vi "Populate Ctrl.vi"(8 "error in (no error)":errorcluster, 11 "FK Field in":refnum<class "FK Field.lvclass">) -> (0 "error out":errorcluster, 3 "FK Field out":refnum<class "FK Field.lvclass">)   [LabVIEW 2020, in "Composed Fields.lvlib" / "FK Field.lvclass"]
uses:
  FK Field.lvclass
  C:/Users/User/Documents/LabVIEW Code/LV-Database-OOP/source/Database OOP/Column Libraries/Column/Composed Column.lvclass
  Ring Ctrl Value Source/Ring Ctrl Value Source.lvclass
  Column/Composed Column.lvclass/Composed Column.ctl
  Composed Columns/Value Source Interface Class/Value Source.lvclass
  Basic Columns/Column Configuration/Basic Column Configuration Class/Column Configuration.lvclass
  Database Libraries/Database Interfaces/Database Interface Class/Database Interface.lvclass
  Column/Composed Column.lvclass
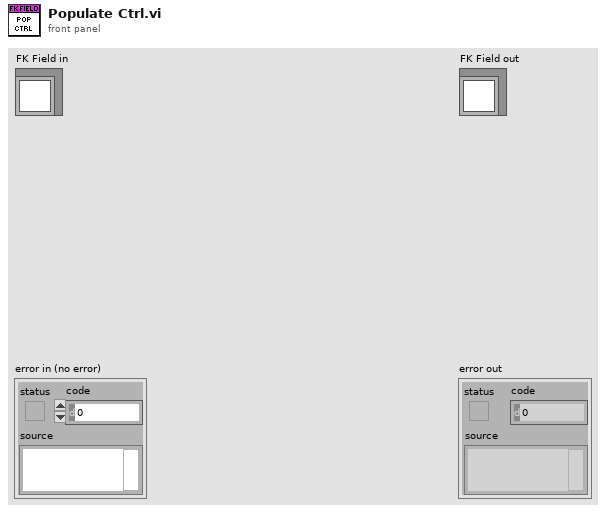
[diagram p1: front panel]
types:
  T1 = typedef "Column Interfaces.lvlib/FK Info.ctl" = cluster{"PK Table":string, "PK Column":string, "PK Display Column":string}
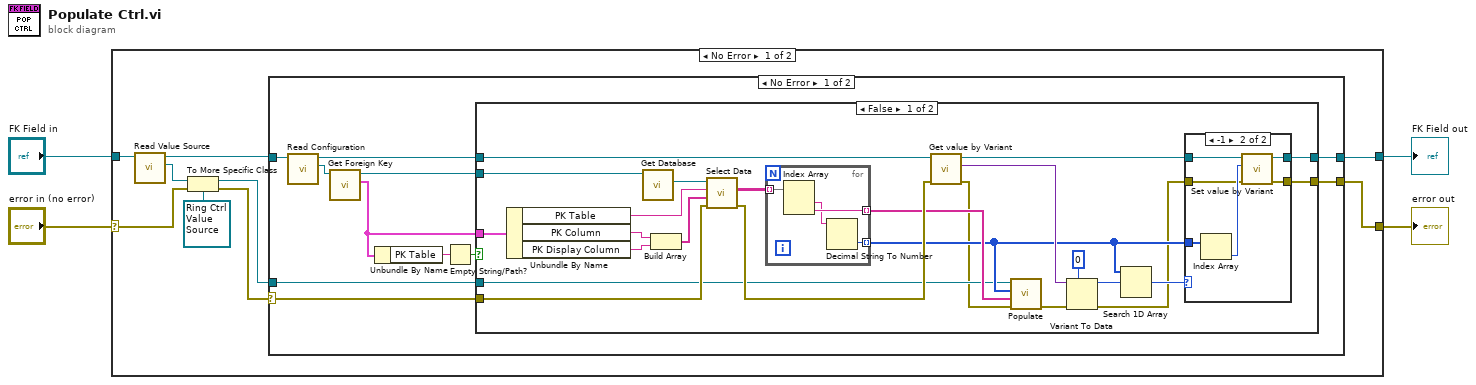
[diagram p0: block diagram]
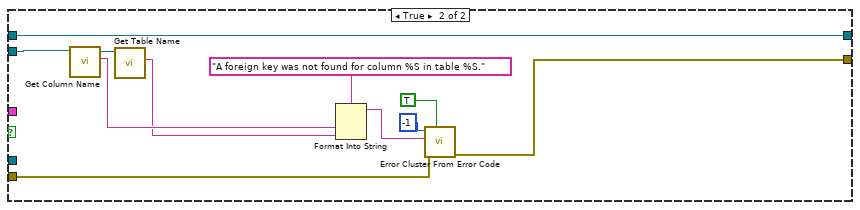
[diagram p3: hidden frame]
diagram:
  n1 = case shown="No Error" "error in (no error)" {
    selector: "error in (no error)" -> [w10 w75]
    tunnel: [w6 w75] -> w2
    tunnel: "FK Field in" -> [w13 w74]
    tunnel: [w5 w74] -> w1
    frame No Error {
      n2 = call "Read Value Source.vi"("Composed Column in"=w13) -> ("Value Source"=w12:refnum<class "Value Source.lvclass">, "Composed Column out"=w9:refnum<class "FK Field.lvclass">)  [unwired: 8 in, 1 out]
      n3 = To More Specific Class(target class=refnum<class "Ring Ctrl Value Source.lvclass"> refnum ("Composed Columns.lvlib:Ring Ctrl Value Source.lvclass"), reference=w12, error in=w10) -> (specific class reference=w7:refnum<class "Ring Ctrl Value Source.lvclass">, error out=w8:errorcluster)
      n4 = case shown="No Error" w8 {
        selector: w8 -> [w23 w72]
        tunnel: [w22 w72] -> w6
        tunnel: w9 -> [w17 w73]
        tunnel: [w21 w73] -> w5
        tunnel: w7 -> [w14 _]
        frame No Error {
          n5 = call "Read Configuration.vi"("Composed Column in"=w17) -> ("Column Interfaces.lvlib:Column Configuration.lvclass"=w15:refnum<class "Column Configuration.lvclass">, "Composed Column out"=w16:refnum<class "FK Field.lvclass">)  [unwired: 8 in, 1 out]
          n6 = call-dynamic "Get Foreign Key.vi"("Basic Column Configuration in"=w15) -> ("FK Info"=w20:T1, "Basic Column Configuration out"=w24:refnum<class "Column Configuration.lvclass">)  [unwired: 7 in, 2 out]
          n7 = Unbundle By Name(w20) -> ("PK Table"=w19:string)
          n8 = Empty String/Path?(string/path=w19) -> (empty?=w18:bool)
          n9 = case shown="False" w18 {
            tunnel: w24 -> [w48 w62]
            tunnel: w23 -> [w42 w64]
            tunnel: [w37 w63] -> w22
            tunnel: w16 -> [w36 w61]
            tunnel: [w33 w61] -> w21
            tunnel: w20 -> [w32 _]
            tunnel: w14 -> [w28 _]
            frame False {
              n10 = Unbundle By Name(w32) -> ("PK Table"=w44:string, "PK Column"=w46:string, "PK Display Column"=w45:string)
              n11 = call-dynamic "Get Database.vi"("Basic Column Configuration in"=w48) -> ("Database"=w47:refnum<class "Database Interface.lvclass">)  [unwired: 8 in, 2 out]
              n12 = Build Array(w46, w45) -> (w43:string[])
              n13 = call-dynamic "Select Data.vi"("error in (no error)"=w42, "Columns"=w43, "Table"=w44, "Database Interface in"=w47) -> ("error out"=w35:errorcluster, "Data"=w41:string[][])  [unwired: 5 in, 1 out]
              n14 = for {
                tunnel: w41 -> [w60] mode=indexing
                tunnel: [w59] -> w30 mode=indexing
                tunnel: [w57] -> w29 mode=indexing
                n15 = Index Array(array=w60) -> (element #1=w58:string, element #2=w59:string)  [unwired: 2 in]
                n16 = Decimal String To Number(string=w58) -> (number=w57:i32)  [unwired: 2 in, 1 out]
              }
              n17 = call-dynamic "Get value by Variant.vi"("error in (no error)"=w35, "Column in"=w36) -> ("error out"=w27:errorcluster, "Variant"=w34:variant, "Column out"=w31:refnum<class "FK Field.lvclass">)  [unwired: 6 in, 1 out]
              n18 = call-dynamic "Populate.vi"("error in (no error)"=w27, "Display Text Array"=w30, "Values Array"=w29, "Ring Ctrl Value Source in"=w28) -> ("error out"=w26:errorcluster)  [unwired: 6 in, 1 out]
              n19 = Variant To Data(error in=w26, type=0, Variant=w34) -> (data=w39:i32, error out=w25:errorcluster)
              n20 = Search 1D Array(1D array=w29, element=w39) -> (index of element=w38:i32)  [unwired: 1 in]
              n21 = case shown="-1" w38 {
                tunnel: w29 -> [_ w56]
                tunnel: w25 -> [w50 w52]
                tunnel: [w50 w51] -> w37
                tunnel: w31 -> [w49 w55]
                tunnel: [w49 w54] -> w33
                frame 0, Default {
                }
                frame -1 {
                  n22 = Index Array(array=w56) -> (element=w53:i32)  [unwired: 1 in]
                  n23 = call-dynamic "Set value by Variant.vi"("error in (no error)"=w52, "Variant"=w53, "Column in"=w55) -> ("error out"=w51:errorcluster, "Column out"=w54:refnum<class "FK Field.lvclass">)  [unwired: 7 in]
                }
              }
            }
            frame True {
              n24 = call-dynamic "Get Column Name.vi"("Basic Column Configuration in"=w62) -> ("Column Name"=w69:string, "Basic Column Configuration out"=w70:refnum<class "Column Configuration.lvclass">)  [unwired: 8 in, 1 out]
              n25 = call-dynamic "Get Table Name.vi"("Basic Column Configuration in"=w70) -> ("Table Name"=w68:string)  [unwired: 8 in, 2 out]
              n26 = Format Into String(format string="A foreign key was not found for column %S in table %S.", w69, w68) -> (resulting string=w67:string)  [unwired: 2 in, 1 out]
              n27 = call <vilib>:"Error Cluster From Error Code.vi"("show call chain? (False)"=TRUE, "error in (no error)"=w64, "error message (\"\")"=w67, "error code (0)"=-1) -> ("error out"=w63:errorcluster)  [unwired: 5 in]
            }
          }
        }
        frame Error {
        }
      }
    }
    frame Error {
    }
  }
  "error out" <- w2
  "FK Field out" <- w1
